vi "EnumReadButton.vi"(5 "Button":T1(ring)) -> (2 "Pressed?":bool)   [LabVIEW 2010, in "FTC.lvlib" / "Remote Interface.lvlib"]
uses:
  Remote Interface.lvlib
  Components/Components.lvlib
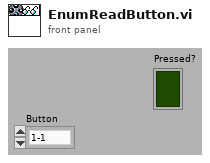
[diagram p1: front panel]
types:
  T1 = enum16{"1-1", "1-2", "1-3", "1-4", "1-5", "1-6", "1-7", "1-8", "1-9", "1-10", "1-11", "1-12", "2-1", "2-2", "2-3", "2-4", "2-5", "2-6", "2-7", "2-8", "2-9", "2-10", "2-11", "2-12", "NXT-L", "NXT-R", "NXT-E", "1-U", "1-UR", "1-R", "1-DR", "1-D", "1-DL", "1-L", "1-UL", "2-U", "2-UR", "2-R", "2-DR", "2-D", "2-DL", "2-L", "2-UL"}
  T2 = typedef "CRef.lvlib/I32 CReference.ctl" = cluster{"Generic CRef Address":u16, "Type":enum8{"Null", "Boolean", "U8", "I8", "U16", "I16", "U32", "I32", "U64", "I64", "Single", "Double", "Extended", "CSG", "CDB", "CXT", "Invalid Def", "U8(Def)", "I8(Def)", "U16(Def)", "I16(Def)", "U32(Def)", "I32(Def)"}}
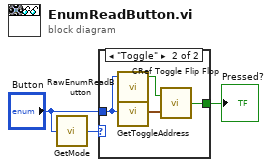
[diagram p0: block diagram]
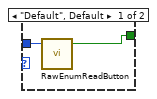
[diagram p2: hidden frame]
diagram:
  n1 = call "GetMode.vi"("Button"="Button") -> ("Mode"=w3:enum16{"Default", "Toggle"})
  n2 = case shown="\"Toggle\"" w3 {
    tunnel: "Button" -> [w4 w8]
    tunnel: [w5 w7] -> w2
    frame "Default", Default {
      n3 = call "RawEnumReadButton.vi"("Button"=w4) -> ("Pressed?"=w5:bool)  [unwired: 4 in]
    }
    frame "Toggle" {
      n4 = call "RawEnumReadButton.vi"("Button"=w8) -> ("Pressed?"=w9:bool)  [unwired: 4 in]
      n5 = call "GetToggleAddress.vi"("Button"=w8) -> ("Address"=w6:T2)
      n6 = call "CRef Toggle Flip Flop.vi"("CRef I32 Address"=w6, "Input"=w9) -> ("Output"=w7:bool)
    }
  }
  "Pressed?" <- w2
